vi "XML to Value (not reentrant).vi"(8 "error in (no error)":errorcluster, 9 "Parent Name Path":string[](array[string]), 10 "Value Tree":T1, 11 "Variant in":variant) -> (0 "error out":errorcluster, 3 "Variant out":variant)   [LabVIEW 2018, in "XML Config.lvlib"]
uses:
  XML Config.lvlib
  <userlib>/_OpenG.lib/lvdata/lvdata.llb/Type Descriptor Enumeration__ogtk.ctl
panel:
  out "name path":string[](array[string])
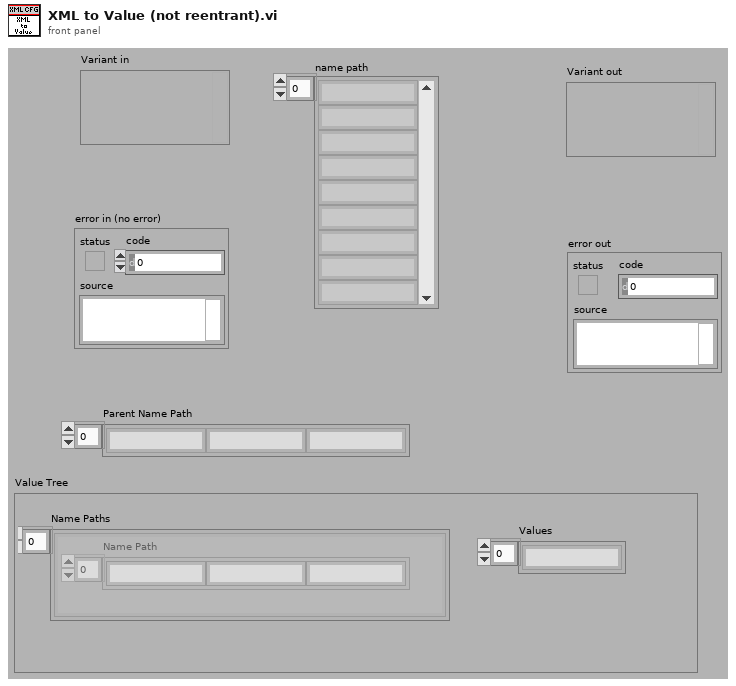
[diagram p1: front panel]
types:
  T1 = cluster{"Name Paths":cluster{"Name Path":string[]}[], "Values":string[]}
  T2 = typedef "Type Descriptor Enumeration__ogtk.ctl" = enum8{"<Null>", "I8", "I16", "I32", "I64", "U8", "U16", "U32", "U64", "SGL", "DBL", "EXT", "CSG", "CDB", "CXT", "0x0F", "0x10", "0x11", "0x12", "0x13", "0x14", "Enum U8", "Enum U16", "Enum U32", "Enum U64", "SGL PQ", "DBL PQ", "EXT PQ", "CSG PQ", "CDB PQ", "CXT PQ", "0x1F", "0x20", "Boolean", "0x22", "0x23", "0x24", "0x25", "0x26", "0x27", "0x28", "0x29", "0x2A", "0x2B", "0x2C", "0x2D", "0x2E", "0x2F", "String", "0x31", "Path", "Pict", "0x34", "0x35", "0x36", "DAQ", "0x38", "0x39", "0x3A", "0x3B", "0x3C", "0x3D", "0x3E", "0x3F", "Array", "0x41", "0x42", "0x43", "0x44", "0x45", "0x46", "0x47", "0x48", "0x49", "0x4A", "0x4B", "0x4C", "0x4D", "0x4E", "0x4F", "Cluster", "0x51", "0x52", "Variant", "Waveform", "0x55", "0x56", "0x57", "0x58", "0x59", "0x5A", "0x5B", "0x5C", "0x5D", "0x5E", "0x5F", "0x60", "0x61", "0x62", "0x63", "0x64", "0x65", "0x66", "0x67", "0x68", "0x69", "0x6A", "0x6B", "0x6C", "0x6D", "0x6E", "0x6F", "Refnum"}
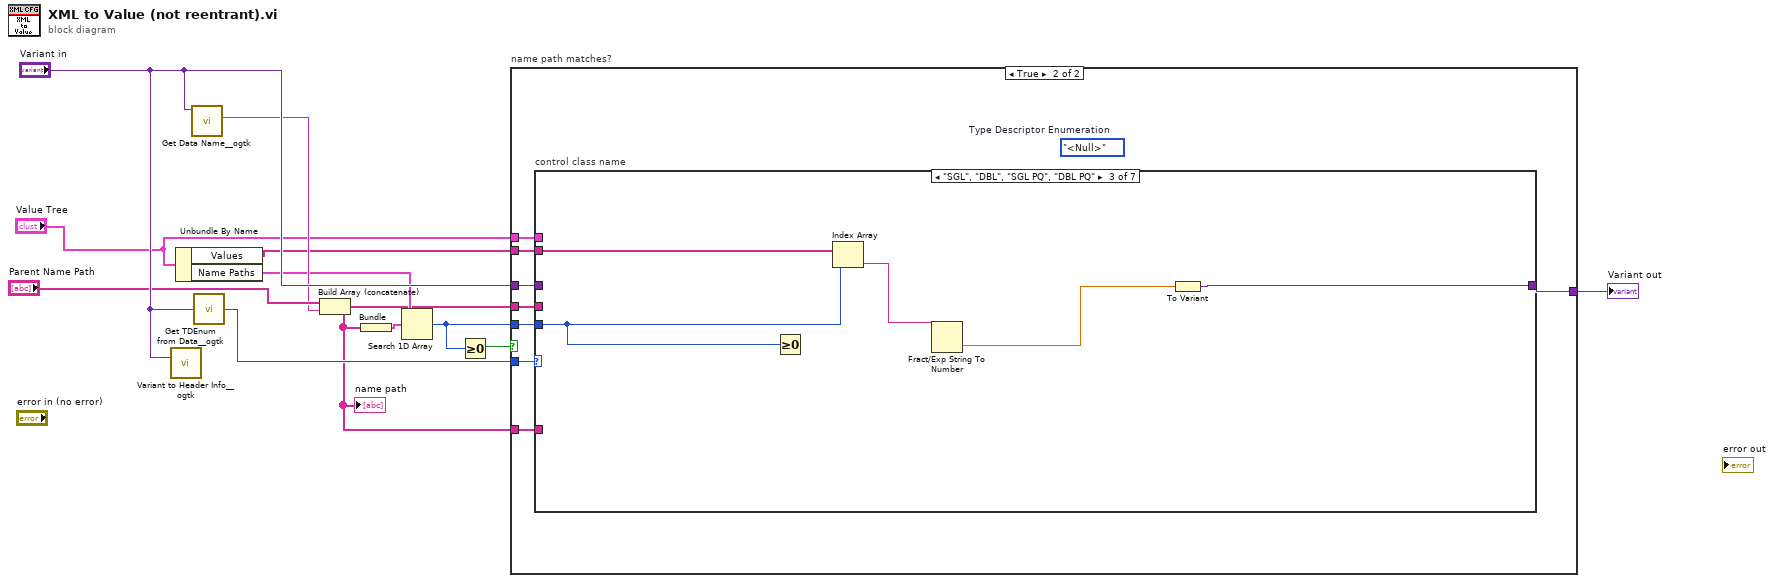
[diagram p0: block diagram]
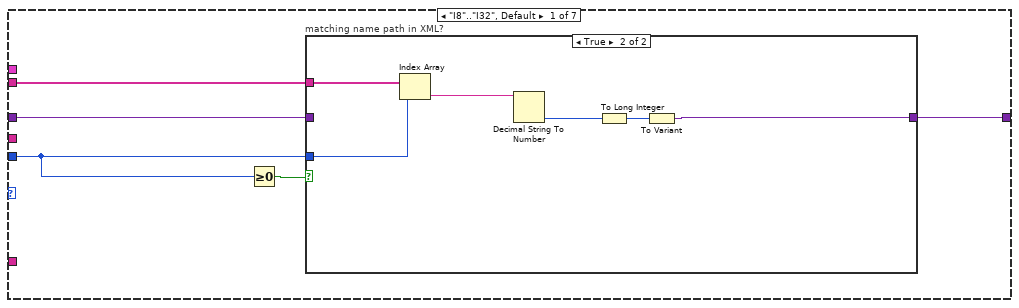
[diagram p3: hidden frame]
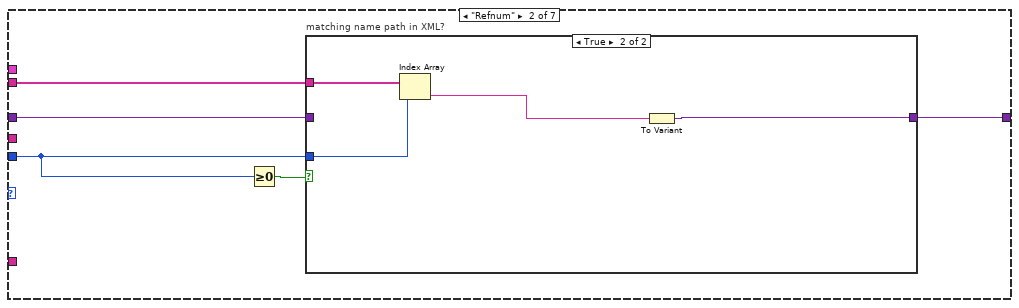
[diagram p5: hidden frame]
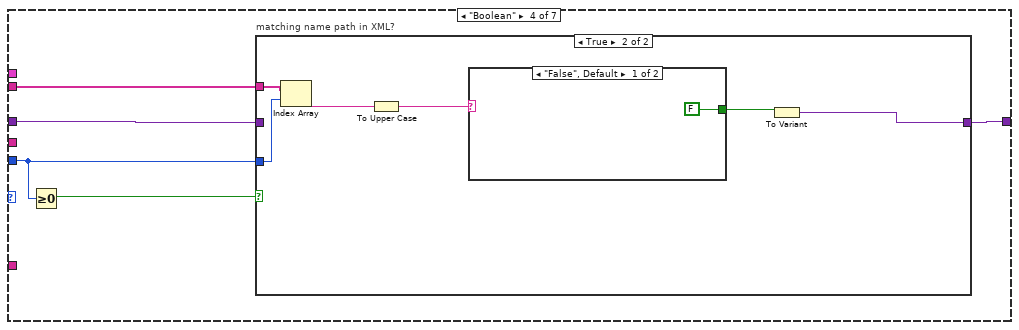
[diagram p7: hidden frame]
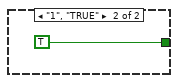
[diagram p9: hidden frame]
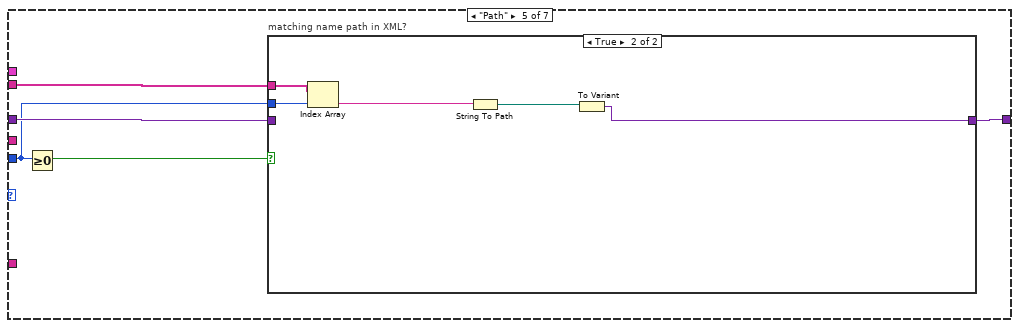
[diagram p10: hidden frame]
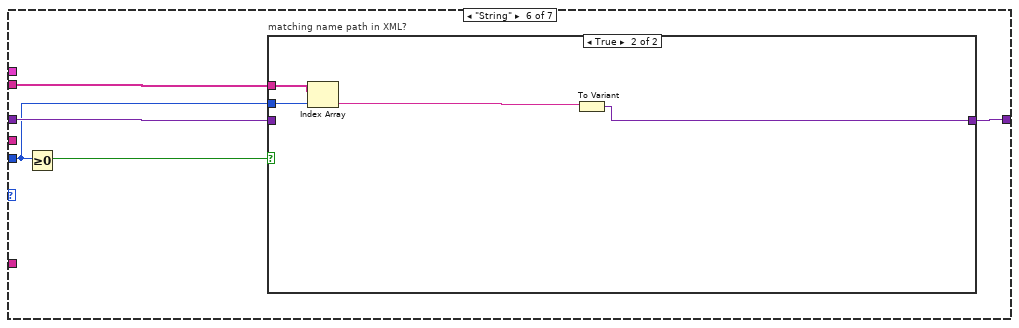
[diagram p12: hidden frame]
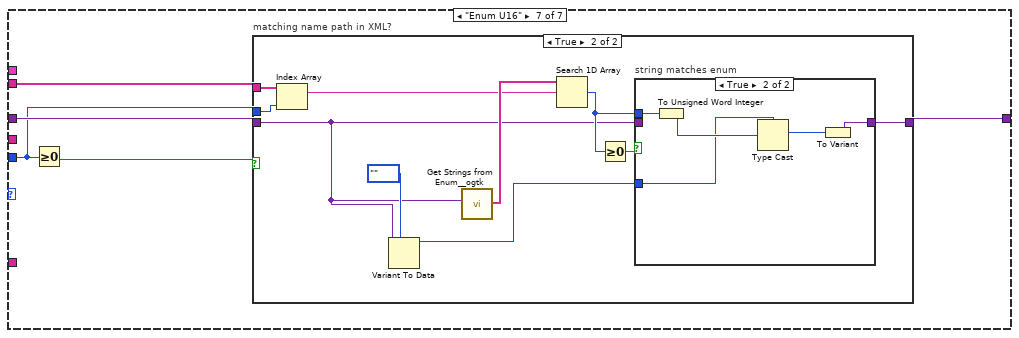
[diagram p14: hidden frame]
diagram:
  n1 = call <userlib>:"Variant to Header Info__ogtk.vi"("Variant"="Variant in") -> ()  [unwired: 3 in, 3 out]
  n2 = Unbundle By Name("Value Tree") -> ("Values"=w6:string[], "Name Paths"=w8:cluster{"Name Path":string[]}[])
  n3 = call <userlib>:"Get Data Name__ogtk.vi"("Data"="Variant in") -> ("Data Name"=w9:string)  [unwired: 8 in, 2 out]
  n4 = call <userlib>:"Get TDEnum from Data__ogtk.vi"("Data"="Variant in") -> ("Type Descriptor Enumeration"=w12:T2)  [unwired: 4 in]
  n5 = Build Array (concatenate)("Parent Name Path", w9) -> (w1:string[])
  "name path" <- w1
  n6 = Bundle(w1) -> (w7:cluster{string[]})  [unwired: 1 in]
  n7 = Search 1D Array(1D array=w8, element=w7) -> (index of element=w3:i32)  [unwired: 1 in]
  n8 = Greater Or Equal To 0?(x=w3) -> (x >= 0?=w2:bool)
  n9 = case "name path matches?" shown="True" w2 {
    tunnel: w12 -> [_ w21]
    tunnel: "Variant in" -> [w13 w20]
    tunnel: w6 -> [_ w19]
    tunnel: [w13 w18] -> w5
    tunnel: w1 -> [_ w17]
    tunnel: "Value Tree" -> [_ w16]
    tunnel: w3 -> [_ w15]
    tunnel: w1 -> [_ w14]
    frame False {
    }
    frame True {
      (unwired) Type_Descriptor_Enumeration__ogtk."<Null>"  # Type Descriptor Enumeration
      n10 = case "control class name" shown="\"SGL\", \"DBL\", \"SGL PQ\", \"DBL PQ\"" w21 {
        tunnel: w20 -> [w26 w38 _ w53 w67 w78 w88]
        tunnel: w19 -> [w25 w37 w48 w52 w64 w75 w87]
        tunnel: w15 -> [w24 w36 w47 w50 w63 w74 w85]
        tunnel: [w22 w34 w46 w49 w65 w76 w84] -> w18
        tunnel: w17 -> [_ _ _ _ _ _ _]
        tunnel: w16 -> [_ _ _ _ _ _ _]
        tunnel: w14 -> [_ _ _ _ _ _ _]
        frame "I8".."I32", Default {
          n11 = Greater Or Equal To 0?(x=w24) -> (x >= 0?=w23:bool)
          n12 = case "matching name path in XML?" shown="True" w23 {
            tunnel: w26 -> [w27 _]
            tunnel: w25 -> [_ w33]
            tunnel: w24 -> [_ w32]
            tunnel: [w27 w28] -> w22
            frame False {
              # "No, use default value"
            }
            frame True {
              n13 = Index Array(array=w33, index=w32) -> (element=w31:string)
              n14 = Decimal String To Number(string=w31) -> (number=w30:i32)  [unwired: 2 in, 1 out]
              n15 = To Long Integer(number=w30) -> (32bit integer=w29:i32)
              n16 = To Variant(anything=w29) -> (Variant=w28:variant)
            }
          }
        }
        frame "Refnum" {
          n17 = Greater Or Equal To 0?(x=w36) -> (x >= 0?=w35:bool)
          n18 = case "matching name path in XML?" shown="True" w35 {
            tunnel: w38 -> [w39 _]
            tunnel: w37 -> [_ w43]
            tunnel: w36 -> [_ w42]
            tunnel: [w39 w41] -> w34
            frame False {
              # "No, use default value"
            }
            frame True {
              n19 = Index Array(array=w43, index=w42) -> (element=w40:string)
              n20 = To Variant(anything=w40) -> (Variant=w41:variant)
            }
          }
        }
        frame "SGL", "DBL", "SGL PQ", "DBL PQ" {
          n21 = Greater Or Equal To 0?(x=w47) -> ()  [unwired: 1 out]
          n22 = Index Array(array=w48, index=w47) -> (element=w45:string)
          n23 = Fract/Exp String To Number(string=w45) -> (number=w44:dbl)  [unwired: 3 in, 1 out]
          n24 = To Variant(anything=w44) -> (Variant=w46:variant)
        }
        frame "Boolean" {
          n25 = Greater Or Equal To 0?(x=w50) -> (x >= 0?=w51:bool)
          n26 = case "matching name path in XML?" shown="True" w51 {
            tunnel: w53 -> [w54 _]
            tunnel: w52 -> [_ w60]
            tunnel: w50 -> [_ w59]
            tunnel: [w54 w55] -> w49
            frame False {
            }
            frame True {
              n27 = Index Array(array=w60, index=w59) -> (element=w58:string)
              n28 = To Upper Case(1:w58) -> (0:w57:string)
              n29 = case shown="\"False\", Default" w57 {
                tunnel: [FALSE TRUE] -> w56
                frame "False", Default {
                }
                frame "1", "TRUE" {
                }
              }
              n30 = To Variant(anything=w56) -> (Variant=w55:variant)
            }
          }
        }
        frame "Path" {
          n31 = Greater Or Equal To 0?(x=w63) -> (x >= 0?=w66:bool)
          n32 = case "matching name path in XML?" shown="True" w66 {
            tunnel: w67 -> [w68 _]
            tunnel: [w68 w69] -> w65
            tunnel: w64 -> [_ w73]
            tunnel: w63 -> [_ w72]
            frame False {
            }
            frame True {
              n33 = Index Array(array=w73, index=w72) -> (element=w71:string)
              n34 = String To Path(string=w71) -> (path=w70:path)
              n35 = To Variant(anything=w70) -> (Variant=w69:variant)
            }
          }
        }
        frame "String" {
          n36 = Greater Or Equal To 0?(x=w74) -> (x >= 0?=w77:bool)
          n37 = case "matching name path in XML?" shown="True" w77 {
            tunnel: w78 -> [w79 _]
            tunnel: [w79 w81] -> w76
            tunnel: w75 -> [_ w83]
            tunnel: w74 -> [_ w82]
            frame False {
            }
            frame True {
              n38 = Index Array(array=w83, index=w82) -> (element=w80:string)
              n39 = To Variant(anything=w80) -> (Variant=w81:variant)
            }
          }
        }
        frame "Enum U16" {
          n40 = Greater Or Equal To 0?(x=w85) -> (x >= 0?=w86:bool)
          n41 = case "matching name path in XML?" shown="True" w86 {
            tunnel: w88 -> [w89 w90]
            tunnel: w87 -> [_ w98]
            tunnel: w85 -> [_ w97]
            tunnel: [w89 w91] -> w84
            frame False {
            }
            frame True {
              n42 = Index Array(array=w98, index=w97) -> (element=w95:string)
              n43 = Variant To Data(type=enum16{""}."", Variant=w90) -> (data=w92:enum16{""})  [unwired: 1 in, 1 out]
              n44 = call <userlib>:"Get Strings from Enum__ogtk.vi"("Enum"=w90) -> ("Enum Strings"=w96:string[])  [unwired: 7 in, 3 out]
              n45 = Search 1D Array(1D array=w96, element=w95) -> (index of element=w94:i32)  [unwired: 1 in]
              n46 = Greater Or Equal To 0?(x=w94) -> (x >= 0?=w93:bool)
              n47 = case "string matches enum" shown="True" w93 {
                tunnel: w94 -> [_ w105]
                tunnel: w92 -> [_ w103]
                tunnel: [w100 w101] -> w91
                tunnel: w90 -> [w100 _]
                frame False {
                }
                frame True {
                  n48 = To Unsigned Word Integer(number=w105) -> (unsigned 16bit integer=w104:u16)
                  n49 = Type Cast(type=w103, x=w104) -> (*(type *) &x=w102:enum16{""})
                  n50 = To Variant(anything=w102) -> (Variant=w101:variant)
                }
              }
            }
          }
        }
      }
    }
  }
  "Variant out" <- w5
